vi "Restore Variable Value.vi"(8 "error in (no error)":errorcluster, 11 "CSM-Static-Variable-Manager in":refnum<class "CSM-Static-Variable-Manager.lvclass">) -> (0 "error out":errorcluster, 3 "CSM-Static-Variable-Manager out":refnum<class "CSM-Static-Variable-Manager.lvclass">)   [LabVIEW 2017, in "INI-Static-Variable-Support.lvlib" / "CSM-Static-Variable-Manager.lvclass"]
uses:
  CSM-Static-Variable-Manager.lvclass
  CSM-Static-Variable-Manager.lvclass/CSM-Static-Variable-Manager.ctl
  LabVIEW-Config/Config.ctl
  LabVIEW-Config/LineToken.ctl
  LabVIEW-Config/LabVIEW-Config.lvlib
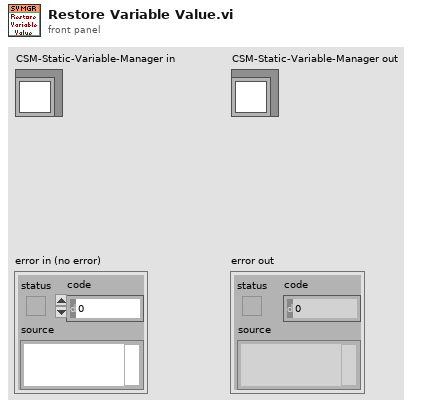
[diagram p1: front panel]
types:
  T1 = typedef "LabVIEW-Config.lvlib/Config.ctl" = cluster{"Path":path, "Lines":string[], "Tokens":T2[], "Modified?":bool}
  T2 = typedef "LabVIEW-Config.lvlib/LineToken.ctl" = enum8{"comment", "section", "key", "more"}
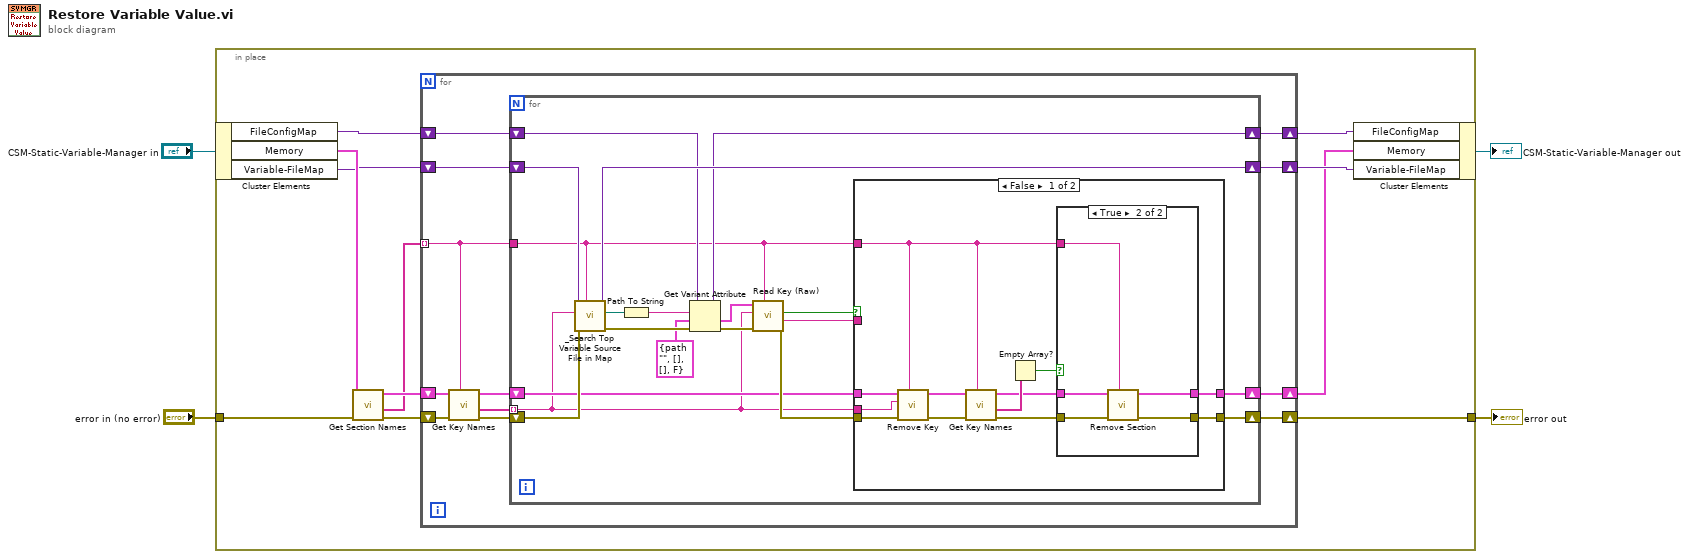
[diagram p0: block diagram]
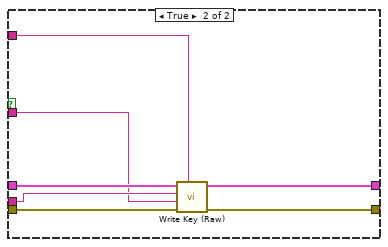
[diagram p3: hidden frame]
diagram:
  n1 = in-place {
    in-place-border: "error in (no error)" -> [w15]
    in-place-border: [w6] -> w1
    n2 = in-place-cluster #1("CSM-Static-Variable-Manager in") -> ("FileConfigMap"=w9:variant, "Memory"=w14:T1, "Variable-FileMap"=w10:variant)
    n3 = call "Get Section Names.vi"("error in (no error)"=w15, "Config in"=w14) -> ("error out"=w12:errorcluster, "Section Names"=w11:string[], "Config out"=w13:T1)  [unwired: 7 in]
    n4 = for {
      shift-right: [w16] -> w6
      shift-left: w12 -> [w26]
      tunnel: w11 -> [w23] mode=indexing
      shift-right: [w17] -> w5
      shift-left: w13 -> [w27]
      shift-right: [w24] -> w7
      shift-left: w10 -> [w25]
      shift-right: [w18] -> w8
      shift-left: w9 -> [w19]
      n5 = call "Get Key Names.vi"("Section Name"=w23, "error in (no error)"=w26, "Config in"=w27) -> ("error out"=w20:errorcluster, "Key Names"=w22:string[], "Config out"=w21:T1)  [unwired: 5 in, 1 out]
      n6 = for {
        tunnel: w23 -> [w32]
        shift-right: [w45] -> w24
        shift-left: w25 -> [w46]
        tunnel: w22 -> [w30] mode=indexing
        shift-right: [w29] -> w17
        shift-left: w21 -> [w33]
        shift-right: [w28] -> w16
        shift-left: w20 -> [w43]
        shift-right: [w38] -> w18
        shift-left: w19 -> [w42]
        n7 = call "_Search Top Variable Source File in Map.vi"("String (section)"=w32, "error in (no error)"=w43, "Content (key)"=w30, "Variable-FileMap"=w46) -> ("error out"=w40:errorcluster, "Top File Path"=w44:path, "Variant"=w45:variant)  [unwired: 5 in]
        n8 = Path To String(path=w44) -> (string=w41:string)
        n9 = Get Variant Attribute(Variant=w42, name=w41, default value (empty Variant)=T1 {"Path"=path "", "Lines"=[], "Tokens"=[], "Modified?"=FALSE} ("Config out"), error in=w40) -> (duplicate Variant=w38:variant, value=w37:T1, error out=w36:errorcluster)  [unwired: 1 out]
        n10 = call "Read Key (Raw).vi"("Section Name"=w32, "error in (no error)"=w36, "Key Name"=w30, "Config in"=w37) -> ("error out"=w34:errorcluster, "Content"=w31:string, "Key Found?"=w35:bool)  [unwired: 4 in, 1 out]
        n11 = case shown="False" w35 {
          tunnel: w34 -> [w57 w70]
          tunnel: w33 -> [w58 w72]
          tunnel: w32 -> [w48 w71]
          tunnel: w31 -> [_ w66]
          tunnel: w30 -> [w47 w67]
          tunnel: [w50 w69] -> w29
          tunnel: [w49 w68] -> w28
          frame False {
            n12 = call "Remove Key.vi"("Section Name"=w48, "error in (no error)"=w57, "Key Name"=w47, "Config in"=w58) -> ("error out"=w55:errorcluster, "Config out"=w56:T1)  [unwired: 5 in, 1 out]
            n13 = call "Get Key Names.vi"("Section Name"=w48, "error in (no error)"=w55, "Config in"=w56) -> ("error out"=w51:errorcluster, "Key Names"=w54:string[], "Config out"=w53:T1)  [unwired: 5 in, 1 out]
            n14 = Empty Array?(array=w54) -> (empty?=w52:bool)
            n15 = case shown="True" w52 {
              tunnel: w53 -> [w60 w65]
              tunnel: w51 -> [w59 w64]
              tunnel: [w60 w63] -> w50
              tunnel: [w59 w62] -> w49
              tunnel: w48 -> [_ w61]
              frame False {
              }
              frame True {
                n16 = call "Remove Section.vi"("Section Name"=w61, "error in (no error)"=w64, "Config in"=w65) -> ("error out"=w62:errorcluster, "Config out"=w63:T1)  [unwired: 6 in, 1 out]
              }
            }
          }
          frame True {
            n17 = call "Write Key (Raw).vi"("Section Name"=w71, "error in (no error)"=w70, "Content"=w66, "Key Name"=w67, "Config in"=w72) -> ("error out"=w68:errorcluster, "Config out"=w69:T1)  [unwired: 4 in, 1 out]
          }
        }
      }
    }
    n18 = in-place-cluster #1("FileConfigMap"=w8, "Memory"=w5, "Variable-FileMap"=w7) -> (→"CSM-Static-Variable-Manager out":refnum<class "CSM-Static-Variable-Manager.lvclass">)
  }
  "error out" <- w1
